vi "calib_T_or_F.vi"(8 "Calibrate":bool, 10 "already calibrated IN":bool) -> (2 "already calibrated OUT":bool)   [LabVIEW 2013]
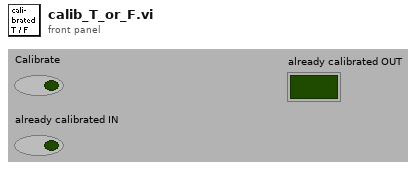
[diagram p1: front panel]
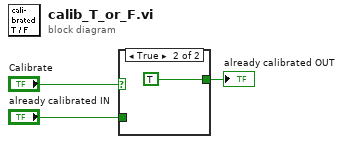
[diagram p0: block diagram]
diagram:
  n1 = case shown="True" "Calibrate" {
    tunnel: [w4 TRUE] -> w2
    tunnel: "already calibrated IN" -> [w4 _]
    frame False {
    }
    frame True {
    }
  }
  "already calibrated OUT" <- w2
